vi "Read Test Queues.vi"(8 "error in (no error)":errorcluster, 11 "Generator in":refnum<class "Generator.lvclass">) -> (0 "error out":errorcluster, 1 "result?":bool, 2 "waveforms":T1, 3 "Generator out":refnum<class "Generator.lvclass">)   [LabVIEW 2019, in "Generator.lvclass"]
uses:
  Generator.lvclass
  typedefs/Waveforms--Cluster.ctl
  Generator.lvclass/Generator.ctl
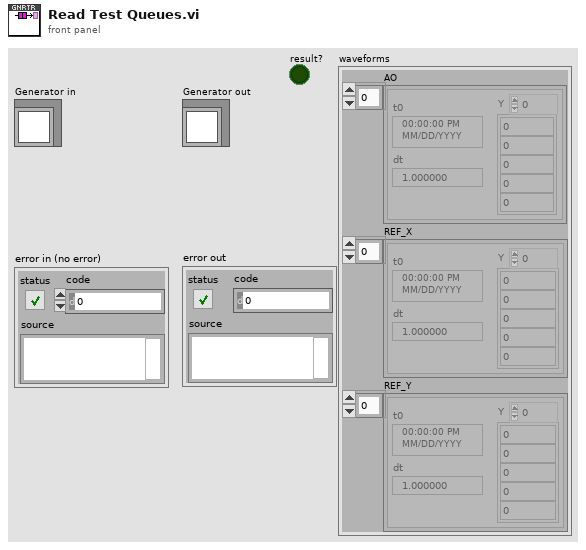
[diagram p1: front panel]
types:
  T1 = typedef "Generator.lvclass/Waveforms--Cluster.ctl" = cluster{"AO":waveform(dbl)[], "REF_X":waveform(dbl)[], "REF_Y":waveform(dbl)[]}
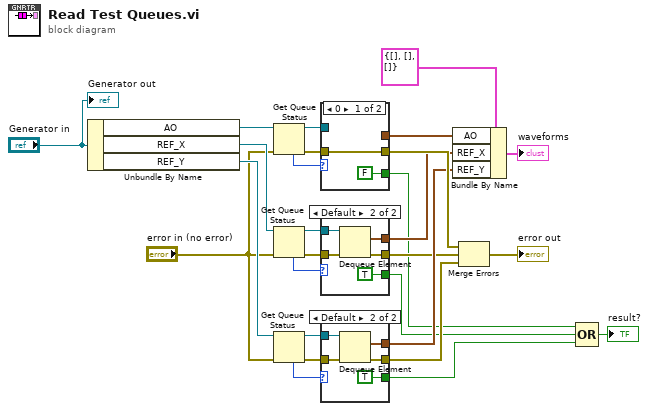
[diagram p0: block diagram]
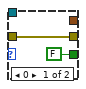
[diagram p2: hidden frame]
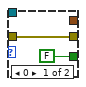
[diagram p3: hidden frame]
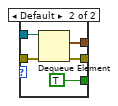
[diagram p4: hidden frame]
diagram:
  n1 = Unbundle By Name("Generator in") -> ("AO"=w19:refnum<queue>, "REF_X"=w20:refnum<queue>, "REF_Y"=w21:refnum<queue>)
  n2 = Get Queue Status(queue=w19, error in (no error)="error in (no error)") -> (queue out=w18:refnum<queue>, error out=w16:errorcluster, # elements in queue=w15:i32)  [unwired: 1 in, 5 out]
  n3 = Get Queue Status(queue=w20, error in (no error)="error in (no error)") -> (queue out=w6:refnum<queue>, error out=w7:errorcluster, # elements in queue=w5:i32)  [unwired: 1 in, 5 out]
  n4 = Get Queue Status(queue=w21, error in (no error)="error in (no error)") -> (queue out=w14:refnum<queue>, error out=w12:errorcluster, # elements in queue=w13:i32)  [unwired: 1 in, 5 out]
  n5 = case shown="0" w15 {
    tunnel: [w29 w34] -> w26
    tunnel: [_ w33] -> w23
    tunnel: w18 -> [_ w32]
    tunnel: w16 -> [w29 w31]
    tunnel: [FALSE TRUE] -> w4
    frame 0 {
    }
    frame Default {
      n6 = Dequeue Element(queue=w32, error in (no error)=w31) -> (element=w33:waveform(dbl)[], error out=w34:errorcluster)  [unwired: 1 in, 2 out]
    }
  }
  n7 = case shown="Default" w5 {
    tunnel: [w36 w41] -> w9
    tunnel: [_ w40] -> w8
    tunnel: w6 -> [_ w39]
    tunnel: w7 -> [w36 w38]
    tunnel: [FALSE TRUE] -> w3
    frame 0 {
    }
    frame Default {
      n8 = Dequeue Element(queue=w39, error in (no error)=w38) -> (element=w40:waveform(dbl)[], error out=w41:errorcluster)  [unwired: 1 in, 2 out]
    }
  }
  n9 = case shown="Default" w13 {
    tunnel: [w43 w48] -> w10
    tunnel: [_ w47] -> w11
    tunnel: w14 -> [_ w46]
    tunnel: w12 -> [w43 w45]
    tunnel: [FALSE TRUE] -> w2
    frame 0 {
    }
    frame Default {
      n10 = Dequeue Element(queue=w46, error in (no error)=w45) -> (element=w47:waveform(dbl)[], error out=w48:errorcluster)  [unwired: 1 in, 2 out]
    }
  }
  n11 = Bundle By Name(cluster=T1 {"AO"=[], "REF_X"=[], "REF_Y"=[]} ("Waveforms"), "AO"=w23, "REF_X"=w8, "REF_Y"=w11) -> (→"waveforms":T1)
  n12 = Merge Errors(w26, w9, w10) -> (→"error out":errorcluster)
  n13 = Compound Arithmetic op=OR(w4, w3, w2) -> (→"result?":bool)
  "Generator out" <- "Generator in"
